vi "计算圆心到拟合圆每个点距离.vi"(9 "Fitted Circle":T1, 11 "Img in":T2) -> (0 "缺口数量":i32, 1 "半径在规格范围内点个数":i32, 2 "圆心到边距离":sgl[](graph), 3 "拟合圆的点数满足规格":bool, 5 "有效缺口数量>=2":bool)   [LabVIEW 2014]
uses:
  <vilib>/vision/Measure.llb/Edge Options.ctl
  <vilib>/vision/Measure.llb/Edge Polarity.ctl
  <vilib>/vision/Measure.llb/Edge New.ctl
  <vilib>/vision/Image Controls.llb/IMAQ Image.ctl
  <vilib>/Analysis/baseanly.llb/Mean (DBL).vi
  <vilib>/vision/NI_Vision_Development_Module.lvlib
  <vilib>/Analysis/NI_AALBase.lvlib
panel:
  out "大小":i32
  out "存储缺口位置":cluster{"X":sgl, "Y":sgl}[](array[cluster])
  out "数组 3":bool[][](array[boolean])
  out "数组":bool[](array[boolean])
  out "圆心到边距离 2":sgl[][](graph)
  out "输出数组 2":sgl[](array[numeric])
  out "输出数组":sgl[](array[numeric])
  out "缺口与圆心连线夹角":dbl[](array[numeric])
  out "Edge Information 2":T3[][](array[typedef]) {"Distance (Real-World)" format="%.2f"; "Location (Real-World)"."Y" format="%.2g"; "Location (Real-World)"."X" format="%.2f"; "Noise" format="%.2f"; "Location (Pixel)"."Y" format="%.2g"; "Location (Pixel)"."X" format="%.2f"; "Strength" format="%.2f"; "Distance (Pixel)" format="%.2f"}
  in  "Options":T4={"Edge Polarity"=2, "Kernel Size"=5, "Width"=7, "Minimum Edge Strength"=20.0, "Interpolation Type"=enum."Bilinear Fixed", "Data Processing Method"=enum."Average"} {"Edge Polarity" items=["All Edges", "Rising Edges", "Falling Edges"]; "Minimum Edge Strength" format="%.2f"; "Width" step=2; "Kernel Size" step=2}
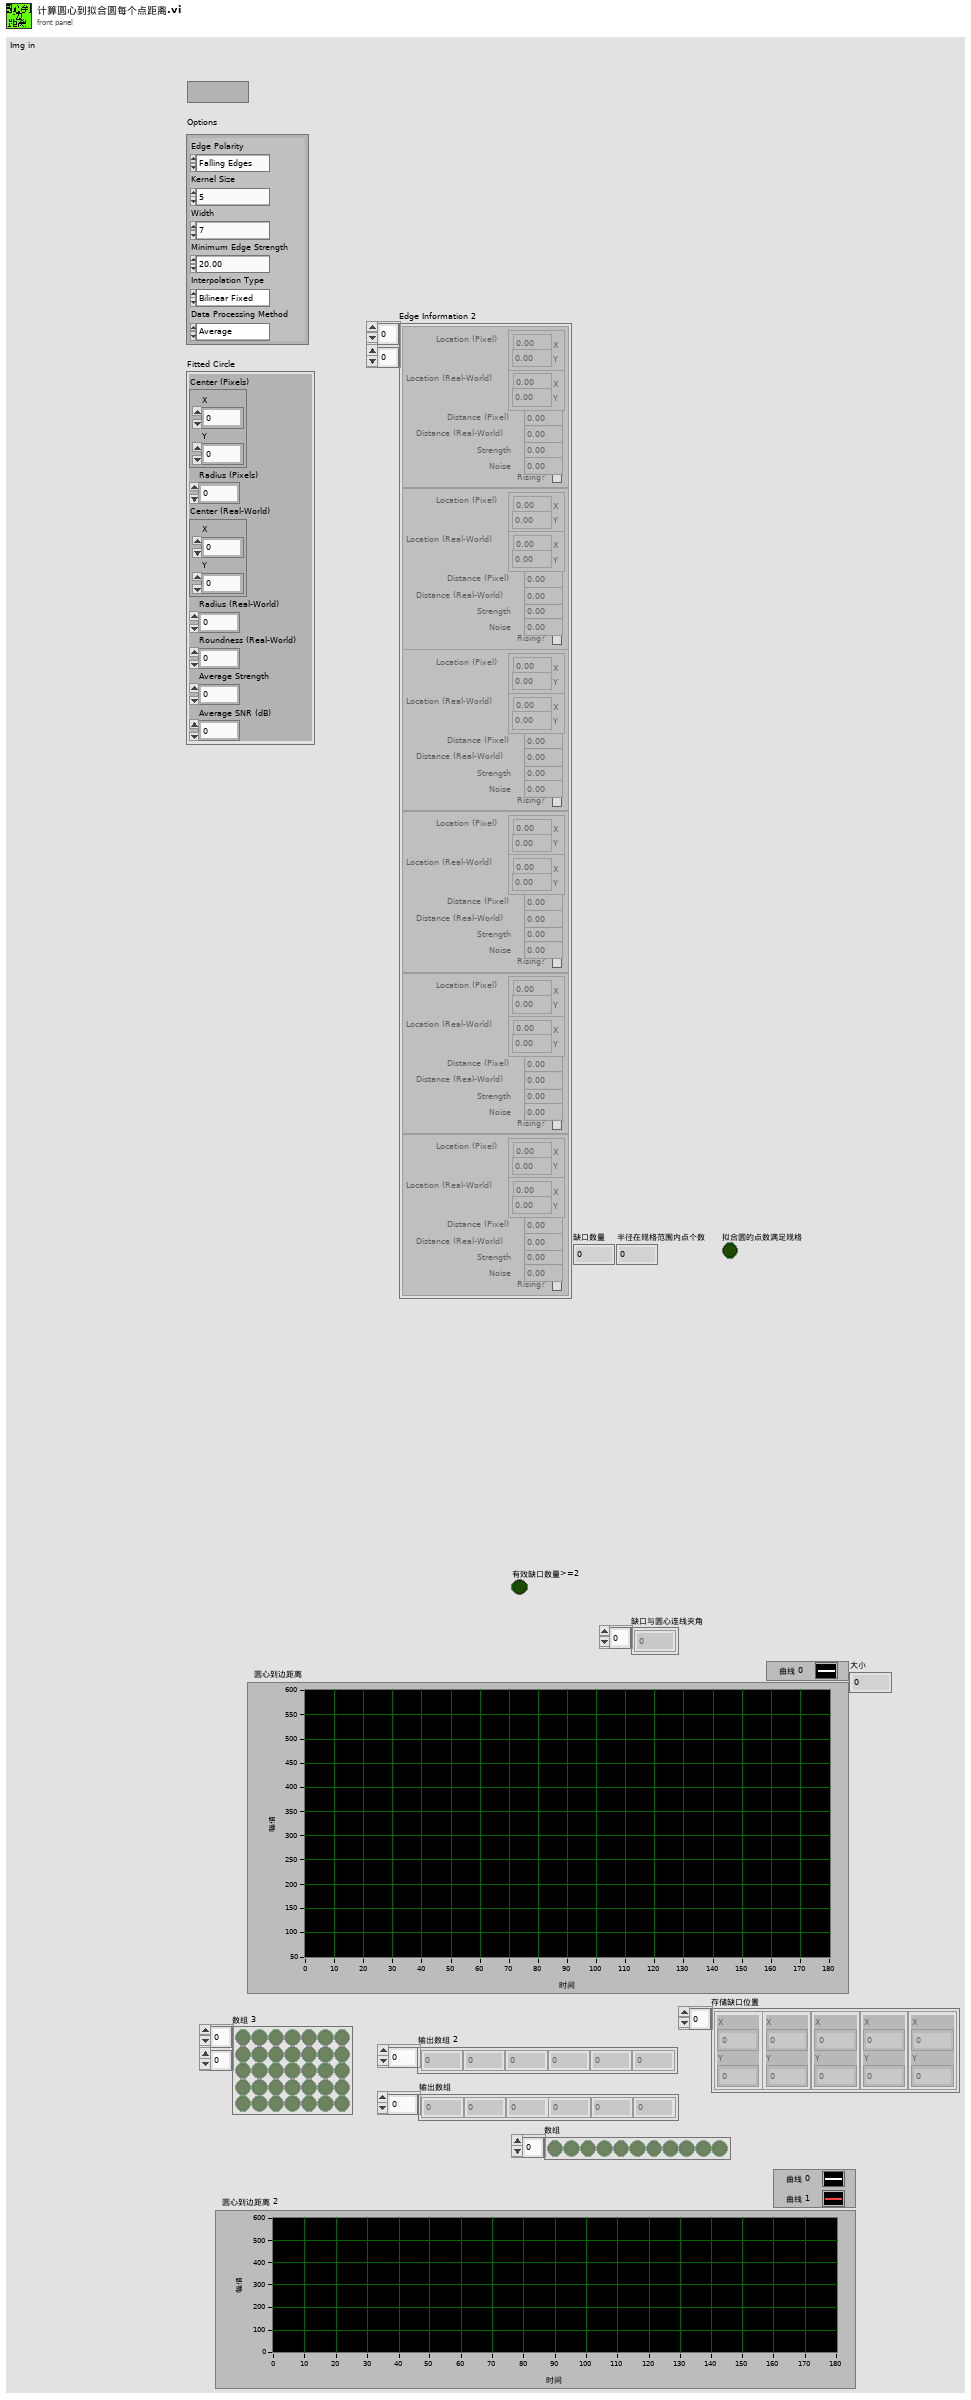
[diagram p1: front panel]
types:
  T1 = cluster{"Center (Pixels)":cluster{"X":sgl, "Y":sgl}, "Radius (Pixels)":dbl, "Center (Real-World)":cluster{"X":sgl, "Y":sgl}, "Radius (Real-World)":dbl, "Roundness (Real-World)":dbl, "Average Strength":dbl, "Average SNR (dB)":dbl}
  T2 = typedef "IMAQ Image.ctl" = refnum<image>
  T3 = typedef "Edge New.ctl" = cluster{"Location (Pixel)":cluster{"X":sgl, "Y":sgl}, "Location (Real-World)":cluster{"X":sgl, "Y":sgl}, "Distance (Pixel)":dbl, "Distance (Real-World)":dbl, "Strength":dbl, "Noise":dbl, "Rising?":bool}
  T4 = typedef "Edge Options.ctl" = cluster{"Edge Polarity":T5, "Kernel Size":u32, "Width":u32, "Minimum Edge Strength":sgl, "Interpolation Type":enum32{"Zero Order", "Bilinear", "Quadratic", "Cubic", "Bilinear Fixed"}, "Data Processing Method":enum32{"Average", "Median"}}
  T5 = typedef "Edge Polarity.ctl" = u32
  T6 = enum16{"Get First Edge", "Get First + Last Edge", "Get All Edges", "Get Best Edge"}
  T7 = typedef "ROI Descriptor" = cluster{"Global Rectangle":i32[], "Contours":cluster{"ID":enum32{"External", "Internal"}, "Type":u32, "Coordinates":i32[]}[]}
  T8 = cluster{"Desired Font (Application)":enum16{"User-specified Font", "Application Font", "System Font", "Dialog Font"}, "[User-specified Font]":cluster{"Font Name":string, "Size":i16, "Strikeout?":bool, "Italic?":bool, "Underline?":bool, "Outline?":bool, "Shadow?":bool, "Bold?":bool, "Rotation Angle":dbl}, "Horizontal Alignment":i16, "Vertical Alignment":i16}
  T9 = cluster{"Center (Pixels)":cluster{"X":sgl, "Y":sgl}, "Center (Pixels)":cluster{"X":sgl, "Y":sgl}}
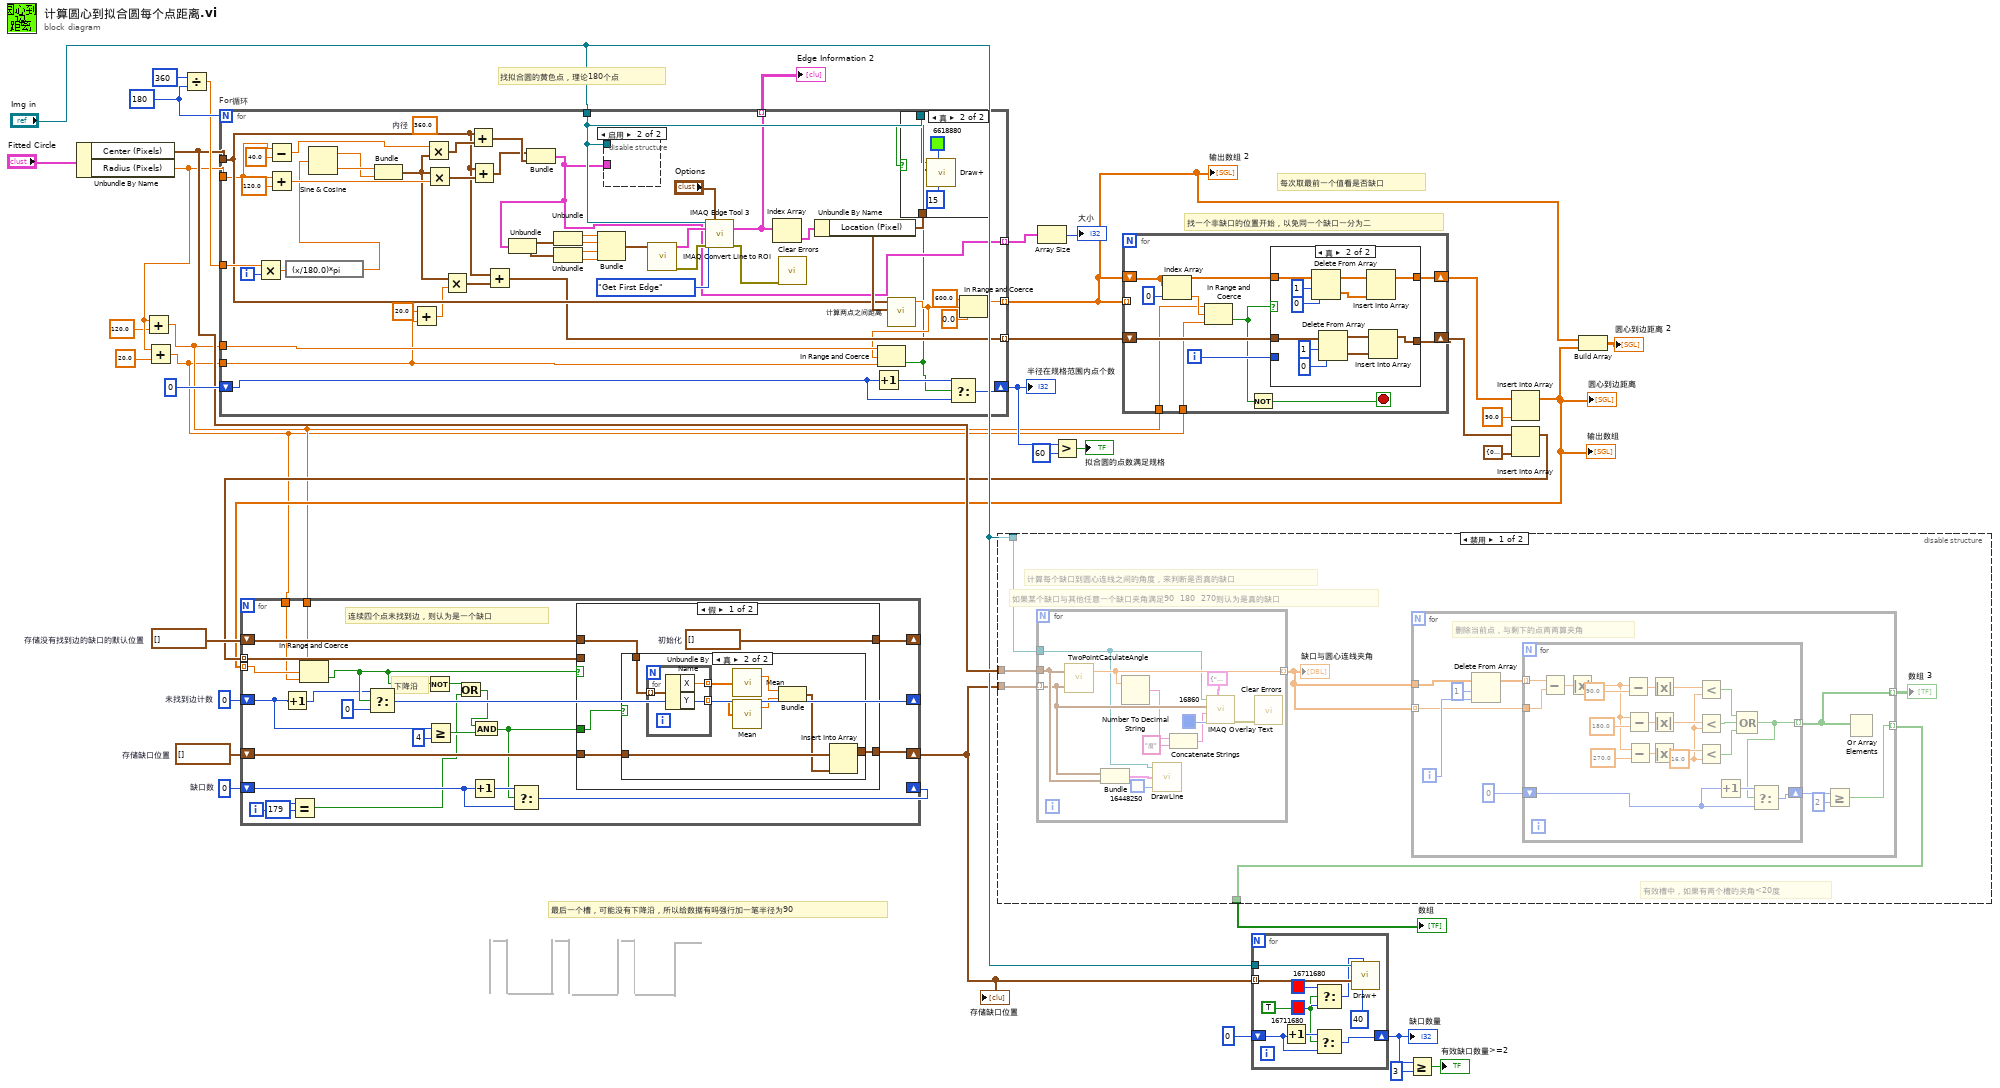
[diagram p0: block diagram]
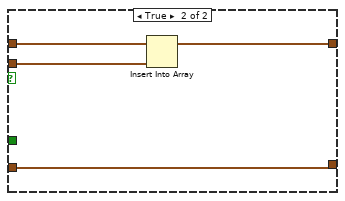
[diagram p5: hidden frame]
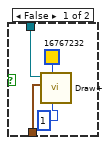
[diagram p6: hidden frame]
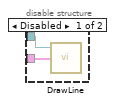
[diagram p7: hidden frame]
diagram:
  w29 = cluster{"X":sgl, "Y":sgl}[] []  # 存储缺口位置
  w30 = cluster{"X":sgl, "Y":sgl}[] []  # 存储没有找到边的缺口的默认位置
  w31 = 0  # 未找到边计数
  w32 = 0  # 缺口数
  w37 = 180
  # "每次取最前一个值看是否缺口"
  # "最后一个槽，可能没有下降沿，所以给数据有吗强行加一笔半径为90"
  # "找拟合圆的黄色点，理论180个点"
  # "找一个非缺口的位置开始，以免同一个缺口一分为二"
  n1 = Unbundle By Name("Fitted Circle") -> ("Center (Pixels)"=w24:cluster{"X":sgl, "Y":sgl}, "Radius (Pixels)"=w12:dbl)
  n2 = Add(x=w12, y=120.0) -> (x+y=w2:dbl)
  n3 = Add(x=w12, y=20.0) -> (x+y=w1:dbl)
  n4 = Divide(x=360, y=w37) -> (x/y=w35:dbl)
  n5 = for "For循环" {
    N: w37 -> [_]
    tunnel: w24 -> [w57]
    tunnel: "Img in" -> [w69]
    tunnel: w12 -> [w45]
    tunnel: w35 -> [w66]
    tunnel: [w58] -> w15 mode=indexing
    tunnel: [w61] -> w36 mode=indexing
    tunnel: [w54] -> w20 mode=indexing
    tunnel: w2 -> [w53]
    tunnel: w1 -> [w40]
    shift-right: [w51] -> w27
    shift-left: 0 -> [w50]
    tunnel: [w44] -> w4 mode=indexing
    i -> [w85]
    (unwired) 360.0  # 内径
    n6 = Multiply(x=w66, y=w85) -> (x*y=w80:dbl)
    n7 = Subtract(x=w45, y=40.0) -> (x-y=w46:dbl)
    n8 = Add(x=w45, y=120.0) -> (x+y=w62:dbl)
    n9 = expression code="(x/180.0)*pi" ("degrees to radians")(w80) -> (w48:dbl)
    n10 = Sine & Cosine(0:w48) -> (1:w81:dbl, 2:w82:dbl)
    n11 = Bundle(w82, w81) -> (w55:cluster{dbl, dbl})  [unwired: 1 in]
    n12 = Add(x=20.0, y=w40) -> (x+y=w38:dbl)
    n13 = Multiply(x=w46, y=w55) -> (x*y=w84:cluster{dbl, dbl})
    n14 = Multiply(x=w55, y=w62) -> (x*y=w83:cluster{dbl, dbl})
    n15 = Multiply(x=w55, y=w38) -> (x*y=w56:cluster{dbl, dbl})
    n16 = Add(x=w57, y=w84) -> (x+y=w43:cluster{dbl, dbl})
    n17 = Add(x=w57, y=w83) -> (x+y=w42:cluster{dbl, dbl})
    n18 = Add(x=w57, y=w56) -> (x+y=w54:cluster{dbl, dbl})
    n19 = Bundle(w42, w43) -> (w44:cluster{cluster{dbl, dbl}, cluster{dbl, dbl}})  [unwired: 1 in]
    n20 = Unbundle(w44) -> (w78:cluster{dbl, dbl}, w77:cluster{dbl, dbl})
    n21 = Unbundle(w78) -> (w76:dbl, w75:dbl)
    n22 = Unbundle(w77) -> (w74:dbl, w73:dbl)
    n23 = Bundle(w76, w75, w74, w73) -> (w72:cluster{dbl, dbl, dbl, dbl})  [unwired: 1 in]
    n24 = disable-structure shown="启用" {
      disable-tunnel: w44 -> [w95 _]
      disable-tunnel: w69 -> [w94 _]
      frame Disabled {
        n25 = call "DrawLine.vi"("Edge Points"=w95, "img in"=w94) -> ()  [unwired: 1 in, 1 out]
      }
      frame Enabled {
      }
    }
    n26 = call "IMAQ Convert Line to ROI"("Line"=w72) -> ("error out"=w71:errorcluster, "ROI Descriptor"=w79:T7)  [unwired: 8 in]
    n27 = call "IMAQ Edge Tool 3"("Image"=w69, "Edge Options"="Options", "ROI Descriptor"=w79, "Process"=T6."Get First Edge", "error in (no error)"=w71) -> ("Edge Information"=w61:T3[], "error out"=w68:errorcluster)  [unwired: 6 in, 3 out]
    n28 = Index Array(array=w61) -> (element=w70:T3)  [unwired: 1 in]
    n29 = call <vilib>:"Clear Errors.vi"("error in (no error)"=w68) -> ()  [unwired: 5 in, 2 out]
    n30 = Unbundle By Name(w70) -> ("Location (Pixel)"=w63:cluster{"X":sgl, "Y":sgl})
    n31 = Increment(x=w50) -> (x+1=w52:i32)
    n32 = call "计算两点之间距离.vi"("Location (Pixel)"=w63, "Center (Pixels)"=w57) -> ("两点之间距离"=w49:sgl)  [unwired: 9 in]
    n33 = In Range and Coerce(upper limit=w53, x=w49, lower limit=w40) -> (In Range?=w41:bool)  [unwired: 1 out]
    n34 = case shown="真" w41 {
      tunnel: w69 -> [w88 w93]
      tunnel: w63 -> [w87 w92]
      frame False {
        n35 = call "Draw+.vi"("Width"=1, "Color"=u32 16767232, "input cluster"=w87, "Image In"=w88) -> ()  [unwired: 2 in, 1 out]
      }
      frame True {
        n36 = call "Draw+.vi"("Width"=15, "Color"=u32 6618880, "input cluster"=w92, "Image In"=w93) -> ()  [unwired: 2 in, 1 out]
      }
    }
    n37 = Select(t=w52, s=w41, f=w50) -> (s? t:f=w51:i32)
    n38 = In Range and Coerce(upper limit=sgl 600.0 ("上限"), x=w49, lower limit=sgl 0.0 ("下限")) -> (coerced(x)=w58:sgl)  [unwired: 1 out]
  }
  "Edge Information 2" <- w36
  "半径在规格范围内点个数" <- w27
  "输出数组 2" <- w15
  n39 = Array Size(array=w4) -> (size(s)=→"大小":i32)
  n40 = Greater?(x=w27, y=60) -> (0:→"拟合圆的点数满足规格":bool)
  n41 = for {
    tunnel: w15 -> [_] mode=indexing
    shift-right: [w105] -> w17
    shift-left: w20 -> [w102]
    shift-right: [w104] -> w18
    shift-left: w15 -> [w101]
    tunnel: w2 -> [w98]
    tunnel: w1 -> [w97]
    i -> [w106]
    stop <- w103 stop-if-true
    n42 = Index Array(array=w101, index=0 ("索引")) -> (element=w99:sgl)
    n43 = In Range and Coerce(upper limit=w98, x=w99, lower limit=w97) -> (In Range?=w96:bool)  [unwired: 1 out]
    n44 = Not(x=w96) -> (.not. x?=w103:bool)
    n45 = case shown="真" w96 {
      tunnel: w106 -> [_ _]
      tunnel: w102 -> [w107 w120]
      tunnel: [w107 w119] -> w105
      tunnel: w101 -> [w108 w116]
      tunnel: [w108 w115] -> w104
      frame False {
      }
      frame True {
        n46 = Delete From Array(array=w116, length=1 ("长度"), index=0 ("索引")) -> (deleted portion=w109:sgl[], array with subset deleted=w118:sgl[])
        n47 = Delete From Array(array=w120, length=1 ("长度"), index=0 ("索引")) -> (deleted portion=w110:cluster{dbl, dbl}[], array with subset deleted=w113:cluster{dbl, dbl}[])
        n48 = Insert Into Array ("数组插入")(array=w118, new element=w109) -> (w115:sgl[])  [unwired: 1 in]
        n49 = Insert Into Array ("数组插入")(array=w113, new element=w110) -> (w119:cluster{dbl, dbl}[])  [unwired: 1 in]
      }
    }
  }
  n50 = Insert Into Array(array=w18, new element=sgl 90.0 ("新元素/子数组")) -> (w14:sgl[])  [unwired: 1 in]
  "圆心到边距离" <- w14
  "输出数组" <- w14
  n51 = Insert Into Array(array=w17, new element=cluster{dbl, dbl} {0.0, 0.0} ("新元素/子数组")) -> (w16:cluster{dbl, dbl}[])  [unwired: 1 in]
  n52 = for {
    tunnel: w14 -> [w126] mode=indexing
    shift-right: [w139] -> _
    shift-left: w32 -> [w138]
    shift-right: [w144] -> _
    shift-left: w31 -> [w122]
    tunnel: w16 -> [w136] mode=indexing
    shift-right: [w135] -> _
    shift-left: w30 -> [w137]
    shift-right: [w133] -> w22
    shift-left: w29 -> [w134]
    tunnel: w2 -> [w125]
    tunnel: w1 -> [w124]
    i -> [w127]
    # "下降沿"
    # "连续四个点未找到边，则认为是一个缺口"
    n53 = Increment(x=w122) -> (x+1=w121:i32)
    n54 = Equal?(x=w127, y=179) -> (x = y?=w128:bool)
    n55 = In Range and Coerce(upper limit=w125, x=w126, lower limit=w124) -> (In Range?=w123:bool)  [unwired: 1 out]
    n56 = Select(t=w121, s=w123, f=0) -> (s? t:f=w144:i32)
    n57 = Not(x=w123) -> (.not. x?=w131:bool)
    n58 = Greater Or Equal?(x=w122, y=4) -> (x >= y?=w141:bool)
    n59 = Or(x=w131, y=w128) -> (x .or. y?=w130:bool)
    n60 = Increment(x=w138) -> (x+1=w140:i32)
    n61 = And(x=w130, y=w141) -> (x .and. y?=w132:bool)
    n62 = Select(t=w140, s=w132, f=w138) -> (s? t:f=w139:i32)
    n63 = case shown="假" w123 {
      tunnel: w137 -> [w148 w165]
      tunnel: w136 -> [_ w164]
      tunnel: [w149 w163] -> w135
      tunnel: w134 -> [w147 w162]
      tunnel: w132 -> [w145 _]
      tunnel: [w146 w162] -> w133
      frame False {
        w149 = cluster{"X":sgl, "Y":sgl}[] []  # 初始化
        n64 = case shown="真" w145 {
          tunnel: w148 -> [_ w158]
          tunnel: w147 -> [w150 w153]
          tunnel: [w150 w151] -> w146
          frame False {
          }
          frame True {
            n65 = for {
              tunnel: w158 -> [w161] mode=indexing
              tunnel: [w160] -> w157 mode=indexing
              tunnel: [w159] -> w156 mode=indexing
              n66 = Unbundle By Name(w161) -> ("X"=w160:sgl, "Y"=w159:sgl)
            }
            n67 = call-poly <vilib>:"Mean.vi"("X"=w157) -> ("mean"=w154:dbl)  [unwired: 1 out]
            n68 = call-poly <vilib>:"Mean.vi"("X"=w156) -> ("mean"=w155:dbl)  [unwired: 1 out]
            n69 = Bundle("mean"=w154, "mean"=w155) -> (w152:cluster{"mean":dbl, "mean":dbl})  [unwired: 1 in]
            n70 = Insert Into Array(array=w153, new element=w152) -> (w151:cluster{"X":sgl, "Y":sgl}[])  [unwired: 1 in]
          }
        }
      }
      frame True {
        n71 = Insert Into Array(array=w165, new element=w164) -> (w163:cluster{"X":sgl, "Y":sgl}[])  [unwired: 1 in]
      }
    }
  }
  "存储缺口位置" <- w22
  n72 = disable-structure shown="禁用" {
    disable-tunnel: w24 -> [w171 _]
    disable-tunnel: "Img in" -> [w170 _]
    disable-tunnel: w22 -> [w169 _]
    disable-tunnel: [w167 _] -> w10
    frame Disabled {
      # "有效槽中，如果有两个槽的夹角<20度"
      # "如果某个缺口与其他任意一个缺口夹角满足90  180  270则认为是真的缺口"
      # "计算每个缺口到圆心连线之间的角度，来判断是否真的缺口"
      n73 = for {
        tunnel: w169 -> [w210] mode=indexing
        tunnel: w171 -> [w213]
        tunnel: [w214] -> w168 mode=indexing
        tunnel: w170 -> [w209]
        n74 = call "TwoPointCaculateAngle.vi"("Point 2"=w210, "Point 1"=w213) -> ("deg( «×)"=w214:dbl)  [unwired: 1 out]
        n75 = Bundle("Center (Pixels)"=w210, "Center (Pixels)"=w213) -> (w212:T9)  [unwired: 1 in]
        n76 = Number To Decimal String(number=w214) -> (decimal integer string=w205:string)  [unwired: 1 in]
        n77 = call "DrawLine.vi"("Color"=u32 16448250, "Edge Points"=w212, "img in"=w209) -> ()  [unwired: 1 out]
        n78 = Concatenate Strings(w205, "度" ("字符串")) -> (w204:string)
        n79 = call "IMAQ Overlay Text"("Text Color (black)"=u32 16860 ("字体颜色"), "Font, Size & Style"=T8 {"Desired Font (Application)"=enum."User-specified Font", "[User-specified Font]"={"Font Name"="", "Size"=20, "Strikeout?"=FALSE, "Italic?"=FALSE, "Underline?"=FALSE, "Outline?"=FALSE, "Shadow?"=FALSE, "Bold?"=TRUE, "Rotation Angle"=0.0}, "Horizontal Alignment"=0, "Vertical Alignment"=0}, "String"=w204, "Origin"=w210, "Image"=w209) -> ("error out"=w206:errorcluster)  [unwired: 5 in, 1 out]
        n80 = call <vilib>:"Clear Errors.vi"("error in (no error)"=w206) -> ()  [unwired: 5 in, 2 out]
      }
      "缺口与圆心连线夹角" <- w168
      n81 = for {
        tunnel: w168 -> [w177] mode=indexing
        tunnel: [w172] -> w167 mode=indexing
        tunnel: w168 -> [w181]
        tunnel: [w176] -> w166 mode=indexing
        i -> [w180]
        # "删除当前点，与剩下的点两两算夹角"
        n82 = Delete From Array(array=w181, length=1 ("长度"), index=w180) -> (array with subset deleted=w178:dbl[])  [unwired: 1 out]
        n83 = for {
          tunnel: w178 -> [w202] mode=indexing
          tunnel: w177 -> [w201]
          tunnel: [w183] -> w176 mode=indexing
          shift-right: [w184] -> w174
          shift-left: 0 -> [w182]
          w189 = 16.0 ("y")
          n84 = Subtract(x=w202, y=w201) -> (x-y=w200:dbl)
          n85 = Absolute Value(x=w200) -> (abs(x)=w196:dbl)
          n86 = Subtract(x=w196, y=90.0) -> (x-y=w195:dbl)
          n87 = Subtract(x=w196, y=180.0) -> (x-y=w194:dbl)
          n88 = Subtract(x=w196, y=270.0) -> (x-y=w193:dbl)
          n89 = Absolute Value(x=w195) -> (abs(x)=w192:dbl)
          n90 = Absolute Value(x=w194) -> (abs(x)=w191:dbl)
          n91 = Absolute Value(x=w193) -> (abs(x)=w190:dbl)
          n92 = Less?(x=w192, y=w189) -> (x < y?=w188:bool)
          n93 = Less?(x=w191, y=w189) -> (x < y?=w187:bool)
          n94 = Less?(x=w190, y=w189) -> (x < y?=w186:bool)
          n95 = Increment(x=w182) -> (x+1=w185:i32)
          n96 = Compound Arithmetic op=OR(w188, w187, w186) -> (w183:bool)
          n97 = Select(t=w185, s=w183, f=w182) -> (s? t:f=w184:i32)
        }
        n98 = Greater Or Equal?(x=w174, y=2) -> (x >= y?=w172:bool)
        n99 = Or Array Elements(Boolean array=w176) -> ()  [unwired: 1 out]
      }
      "数组 3" <- w166
    }
    frame Enabled {
    }
  }
  "数组" <- w10
  n100 = for {
    tunnel: "Img in" -> [w224]
    tunnel: w22 -> [w223] mode=indexing
    shift-right: [w219] -> w8
    shift-left: 0 -> [w218]
    w216 = TRUE ("s")
    n101 = Increment(x=w218) -> (x+1=w220:i32)
    n102 = Select(t=w220, s=w216, f=w218) -> (s? t:f=w219:i32)
    n103 = Select(t=u32 16711680 ("Color"), s=w216, f=u32 16711680 ("Color")) -> (s? t:f=w217:u32)
    n104 = call "Draw+.vi"("Width"=40, "Color"=w217, "input cluster"=w223, "Image In"=w224) -> ()  [unwired: 2 in, 1 out]
  }
  "缺口数量" <- w8
  n105 = Greater Or Equal?(x=w8, y=3) -> (x >= y?=→"有效缺口数量>=2":bool)
  n106 = Build Array(w15, w14) -> (→"圆心到边距离 2":sgl[][])
